vi "Parse Data JSON.vi"(8 "error in (no error)":errorcluster, 10 "JSON String":string, 11 "Event in":refnum<class "Event.lvclass">) -> (0 "error out":errorcluster, 1 "Typed?":bool, 2 "Typed Message":refnum<class "Response.lvclass">, 3 "Event out":refnum<class "Event.lvclass">)   [LabVIEW 2020, in "obs-websocket.lvlib" / "Event.lvclass"]
uses:
  Event.lvclass
  Response/Response.lvclass
  Event.lvclass/Event.ctl
  <vilib>/JDP Science/JSONtext/JSONtext.lvlib
  b3e34c19-5340-4f6b-83d9-2472b6f48d65.vi
  90894fc4-6fe4-4810-bec3-5b6327a60420.vi
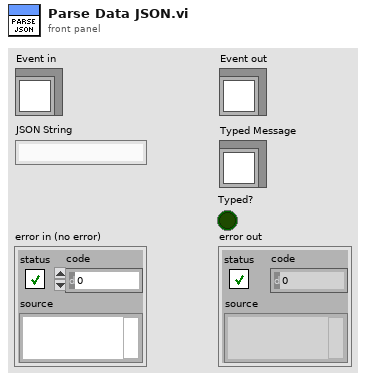
[diagram p1: front panel]
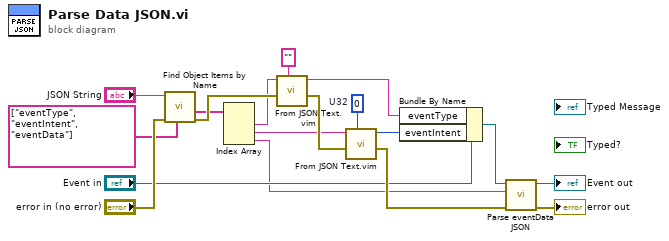
[diagram p0: block diagram]
diagram:
  w4 = u32 0  # U32
  n1 = call <vilib>:"Find Object Items by Name.vi"("Item Names"=string[] ["eventType", "eventIntent", "eventData"] ("Search Keys"), "error in (no error)"="error in (no error)", "JSON"="JSON String") -> ("error out"=w16:errorcluster, "<JSON>"=w8:string[])  [unwired: 6 in, 1 out]
  n2 = Index Array(array=w8) -> (element #1=w7:string, element #2=w5:string, element #3=w3:string)  [unwired: 3 in]
  n3 = call "From JSON Text.vim"("Data Type and Default Value"="", "error in (no error)"=w16, "JSON"=w7) -> ("error out"=w15:errorcluster, "Data out"=w1:string)  [unwired: 7 in]
  n4 = call "From JSON Text.vim"("Data Type and Default Value"=w4, "error in (no error)"=w15, "JSON"=w5) -> ("error out"=w18:errorcluster, "Data out"=w2:u32)  [unwired: 7 in]
  n5 = Bundle By Name(cluster="Event in", "eventType"=w1, "eventIntent"=w2) -> (w13:refnum<class "Event.lvclass">)
  n6 = call-dynamic "Parse eventData JSON.vi"("error in (no error)"=w18, "eventData JSON"=w3, "Event in"=w13) -> ("error out"=→"error out":errorcluster, "Event out"=→"Event out":refnum<class "Event.lvclass">)  [unwired: 7 in]
